vi "Delta T_v2.vi"(8 "Background":dbl[][](array[numeric]), 9 "FrameData":dbl[][][](array[numeric])) -> (0 "FrameData even":dbl[][][](array[numeric]), 1 "FrameData odd":dbl[][][](array[numeric]), 2 "Delta T":dbl[][](array[numeric]), 3 "Delta T over T":dbl[][](array[numeric]))   [LabVIEW 2020]
uses:
  Random subVIs/Control 1.ctl
  <vilib>/Utility/file.llb/Write Delimited Spreadsheet (DBL).vi
panel:
  in  "base path":path
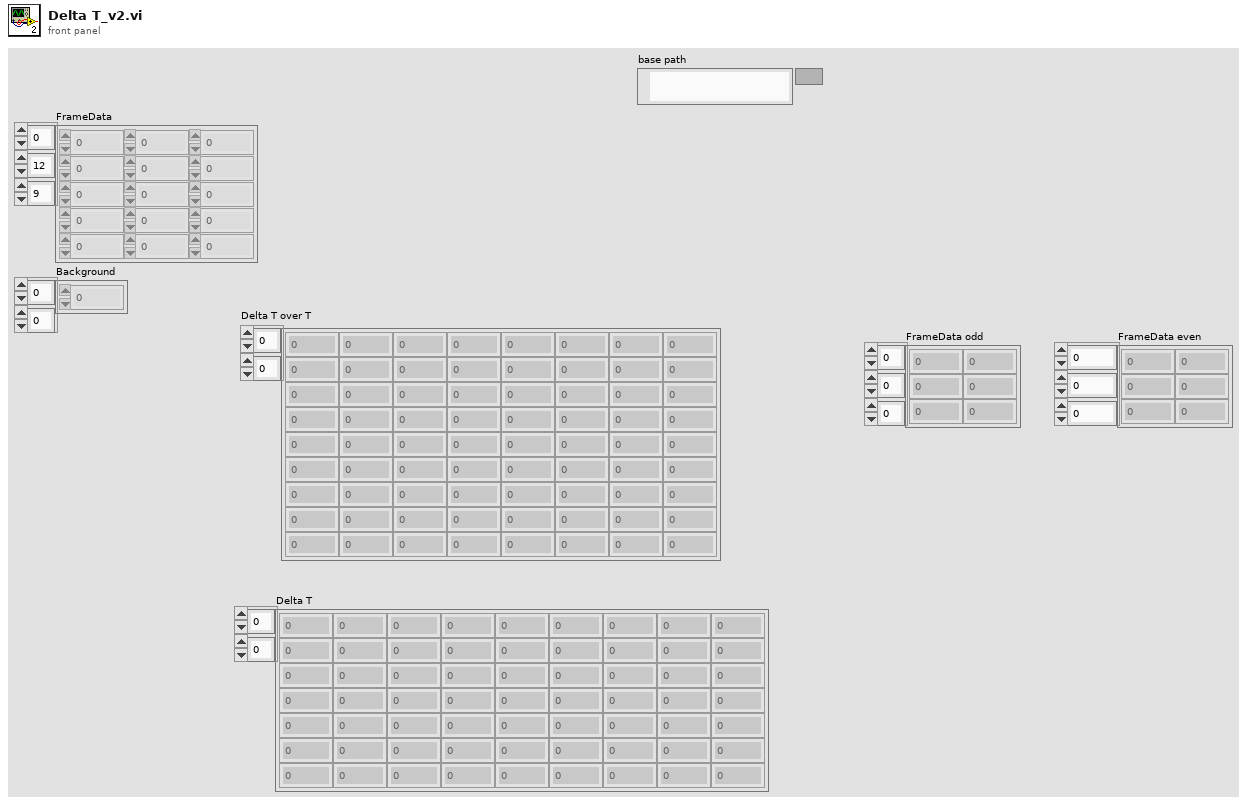
[diagram p1: front panel]
types:
  T1 = enum16{"big-endian, network order", "native, host order", "little-endian"}
  T2 = enum16{"open", "replace", "create", "open or create", "replace or create", "replace or create with confirmation"}
  T3 = typedef "Control 1.ctl" = i32
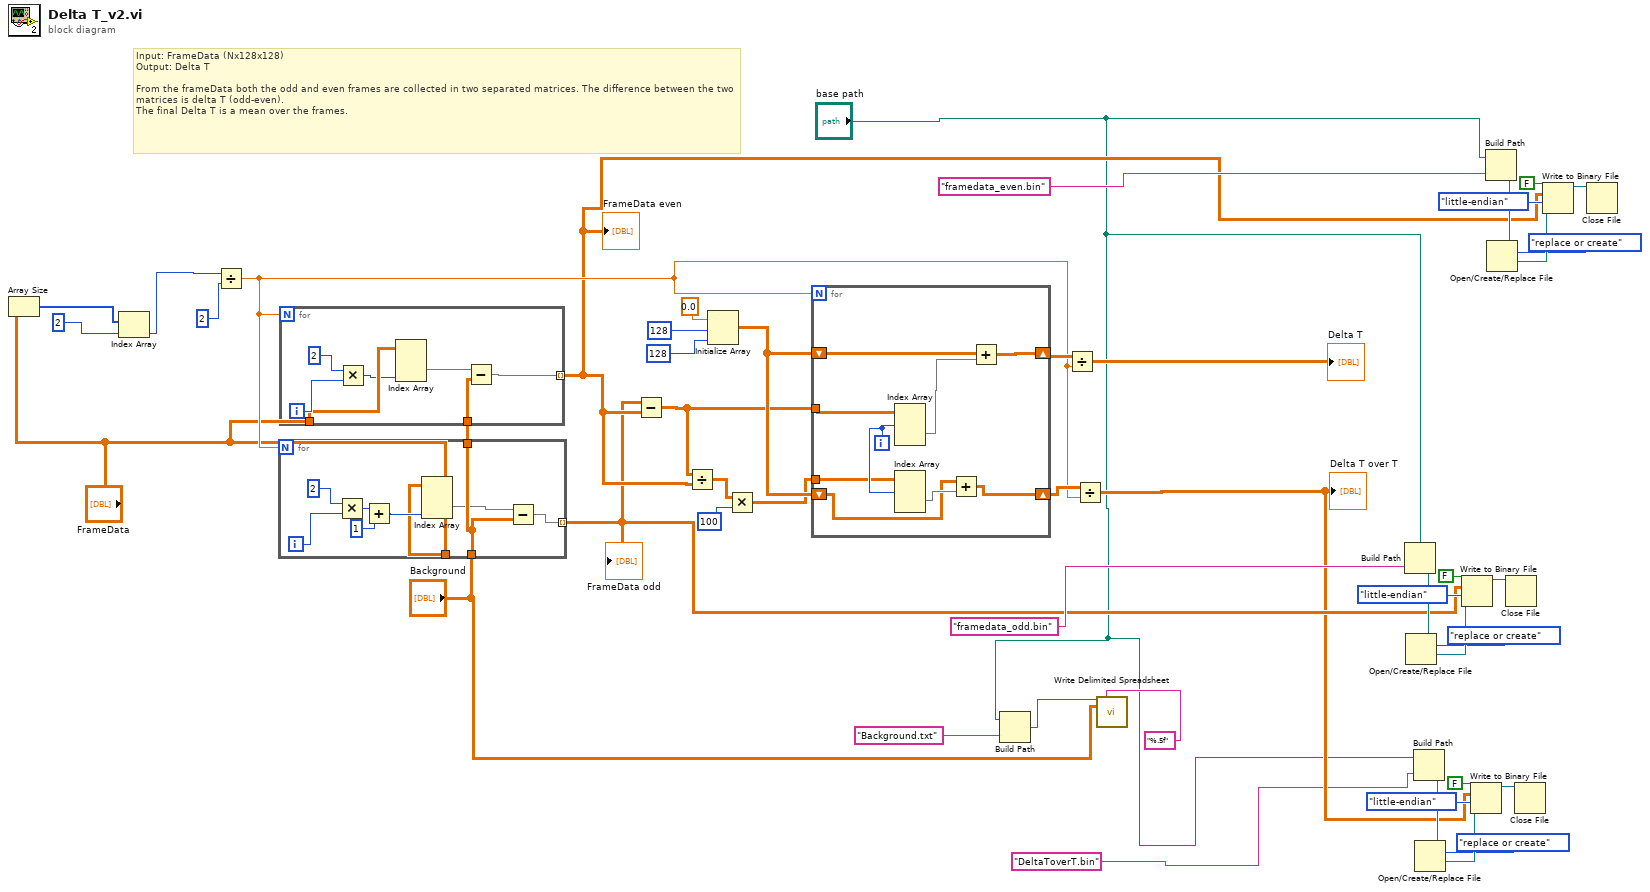
[diagram p0: block diagram]
diagram:
  # "Input: FrameData (Nx128x128)\nOutput: Delta T\n\nFrom the frameData both the odd and even frames are collected in two separated matrices. The difference between the two matrices is delta T (odd-even). \nThe final Delta T is a mean over the frames."
  n1 = Array Size(array="FrameData") -> (size(s)=w41:i32[])
  n2 = Index Array(array=w41, index=2) -> (element=w40:i32)
  n3 = Divide(x=w40, y=T3 2) -> (x/y=w37:dbl)
  n4 = for {
    N: w37 -> [_]
    tunnel: "FrameData" -> [w51]
    tunnel: "Background" -> [w49]
    tunnel: [w50] -> w10 mode=indexing
    tunnel: [w49] -> w34
    i -> [w56]
    n5 = Multiply(x=2, y=w56) -> (x*y=w54:i32)
    n6 = Add(x=w54, y=1) -> (x+y=w52:i32)
    n7 = Index Array(array=w51, index (dim 2)=w52) -> (element=w48:dbl[][])  [unwired: 2 in]
    n8 = Subtract(x=w48, y=w49) -> (x-y=w50:dbl[][])
  }
  "FrameData odd" <- w10
  n9 = for {
    N: w37 -> [_]
    tunnel: [w58] -> w18 mode=indexing
    tunnel: "FrameData" -> [w61]
    tunnel: w34 -> [w59]
    i -> [w63]
    n10 = Multiply(x=2, y=w63) -> (x*y=w60:i32)
    n11 = Index Array(array=w61, index (dim 2)=w60) -> (element=w57:dbl[][])  [unwired: 2 in]
    n12 = Subtract(x=w57, y=w59) -> (x-y=w58:dbl[][])
  }
  "FrameData even" <- w18
  n13 = Subtract(x=w10, y=w18) -> (x-y=w35:dbl[][][])
  n14 = Divide(x=w35, y=w18) -> (x/y=w33:dbl[][][])
  n15 = Initialize Array(0.0 ("element"), 128 ("dimension size"), 128 ("dimension size")) -> (w39:dbl[][])
  n16 = Multiply(x=w33, y=100) -> (x*y=w32:dbl[][][])
  n17 = for {
    N: w37 -> [_]
    tunnel: w35 -> [w72]
    shift-right: [w70] -> w43
    shift-left: w39 -> [w65]
    shift-right: [w67] -> w38
    shift-left: w39 -> [w64]
    tunnel: w32 -> [w66]
    i -> [w69]
    n18 = Index Array(array=w72, index (dim 0)=w69) -> (element=w71:dbl[][])  [unwired: 2 in]
    n19 = Index Array(array=w66, index (dim 0)=w69) -> (element=w68:dbl[][])  [unwired: 2 in]
    n20 = Add(x=w64, y=w68) -> (x+y=w67:dbl[][])
    n21 = Add(x=w65, y=w71) -> (x+y=w70:dbl[][])
  }
  n22 = Build Path(base path="base path", name or relative path="Background.txt" ("string")) -> (appended path=w29:path)
  n23 = Divide(x=w43, y=w37) -> (x/y=→"Delta T":dbl[][])
  n24 = Divide(x=w38, y=w37) -> (x/y=w3:dbl[][])
  "Delta T over T" <- w3
  n25 = call-poly <vilib>:"Write Delimited Spreadsheet.vi"("file path (dialog if empty)"=w29, "format (%.3f)"="%.5f", "2D data"="Background") -> ()  [unwired: 11 in, 2 out]
  n26 = Build Path(base path="base path", name or relative path="framedata_odd.bin" ("string")) -> (appended path=w12:path)
  n27 = Open/Create/Replace File(file path (use dialog)=w12, operation (0:open)=T2."replace or create") -> (refnum out=w17:refnum<file>)  [unwired: 4 in, 2 out]
  n28 = Build Path(base path="base path", name or relative path="DeltaToverT.bin" ("string")) -> (appended path=w4:path)
  n29 = Open/Create/Replace File(file path (use dialog)=w4, operation (0:open)=T2."replace or create") -> (refnum out=w9:refnum<file>)  [unwired: 4 in, 2 out]
  n30 = Write to Binary File(file (use dialog)=w17, data=w10, 5:FALSE ("prepend array or string size? (T)"), 9:T1."little-endian" ("byte order (0:big-endian, network order)")) -> (refnum out=w16:refnum<file>)  [unwired: 2 in, 2 out]
  n31 = Write to Binary File(file (use dialog)=w9, data=w3, 5:FALSE ("prepend array or string size? (T)"), 9:T1."little-endian" ("byte order (0:big-endian, network order)")) -> (refnum out=w8:refnum<file>)  [unwired: 2 in, 2 out]
  n32 = Build Path(base path="base path", name or relative path="framedata_even.bin" ("string")) -> (appended path=w20:path)
  n33 = Open/Create/Replace File(file path (use dialog)=w20, operation (0:open)=T2."replace or create") -> (refnum out=w25:refnum<file>)  [unwired: 4 in, 2 out]
  n34 = Close File(refnum=w16) -> ()  [unwired: 1 in, 2 out]
  n35 = Close File(refnum=w8) -> ()  [unwired: 1 in, 2 out]
  n36 = Write to Binary File(file (use dialog)=w25, data=w18, 5:FALSE ("prepend array or string size? (T)"), 9:T1."little-endian" ("byte order (0:big-endian, network order)")) -> (refnum out=w24:refnum<file>)  [unwired: 2 in, 2 out]
  n37 = Close File(refnum=w24) -> ()  [unwired: 1 in, 2 out]
